vi "MULT_Amostragem_IceMen_FI.vi"(0 "3458A Master":string="22") -> ()   [LabVIEW 2014]
panel:
  out "f":dbl format="%#_8g"
  out "Phase Diff DMM1-DMM2(sec)":dbl[](graph)
  out "FFT":dbl[][](graph)
  out "Phase Diff(sec)":dbl format="%#_10p"
  out "Waveform Graph":dbl[][](graph)
  out "data 2":string
  in  "SLAVE":path=path "C:/Users/diele/Desktop/medição master-slave/SLAVE.txt"
  out "error out 2":errorcluster
  out "OLA EU SOU SLAVE:":string
  in  "3458A Slave":string="3"
  in  "Atraso":i32(ring)=1 items=["", "Inteiro", "Fracionário"]
  in  "Filtro LF":bool
  out "data":string
  out "Abertura (s)":dbl=170.0 min=0.1 max=500.0 step=0.1 format="%#_4g"
  out "V RMS":dbl format="%#_10g"
  out "Delay":dbl=0.10000000149011612 min=0.10000000149011612 max=10000.0 step=0.10000000149011612 format="%.7f"
  out "Harmonicos Medidos":i32
  out "FREQUÊNCIA":dbl format="%#_10g"
  out "Número de Amostras":i32
  out "Intervalo de Amostragem (s)":dbl format="%_10g"
  in  "Número de Harmônicos":i32=50 min=0 max=200 step=1
  out "Iterações":i32
  in  "MASTER":path=path "C:/Users/diele/Desktop/medição master-slave/MASTER.txt"
  in  "NÚMERO DE TRENS DE AMOSTRA":i32=100 min=1 max=1000 step=1
  out "error out":errorcluster
  out "OLA EU SOU MASTER:":string
  # "Aquisição de sinais em baixa frequência através de amostragem digital."
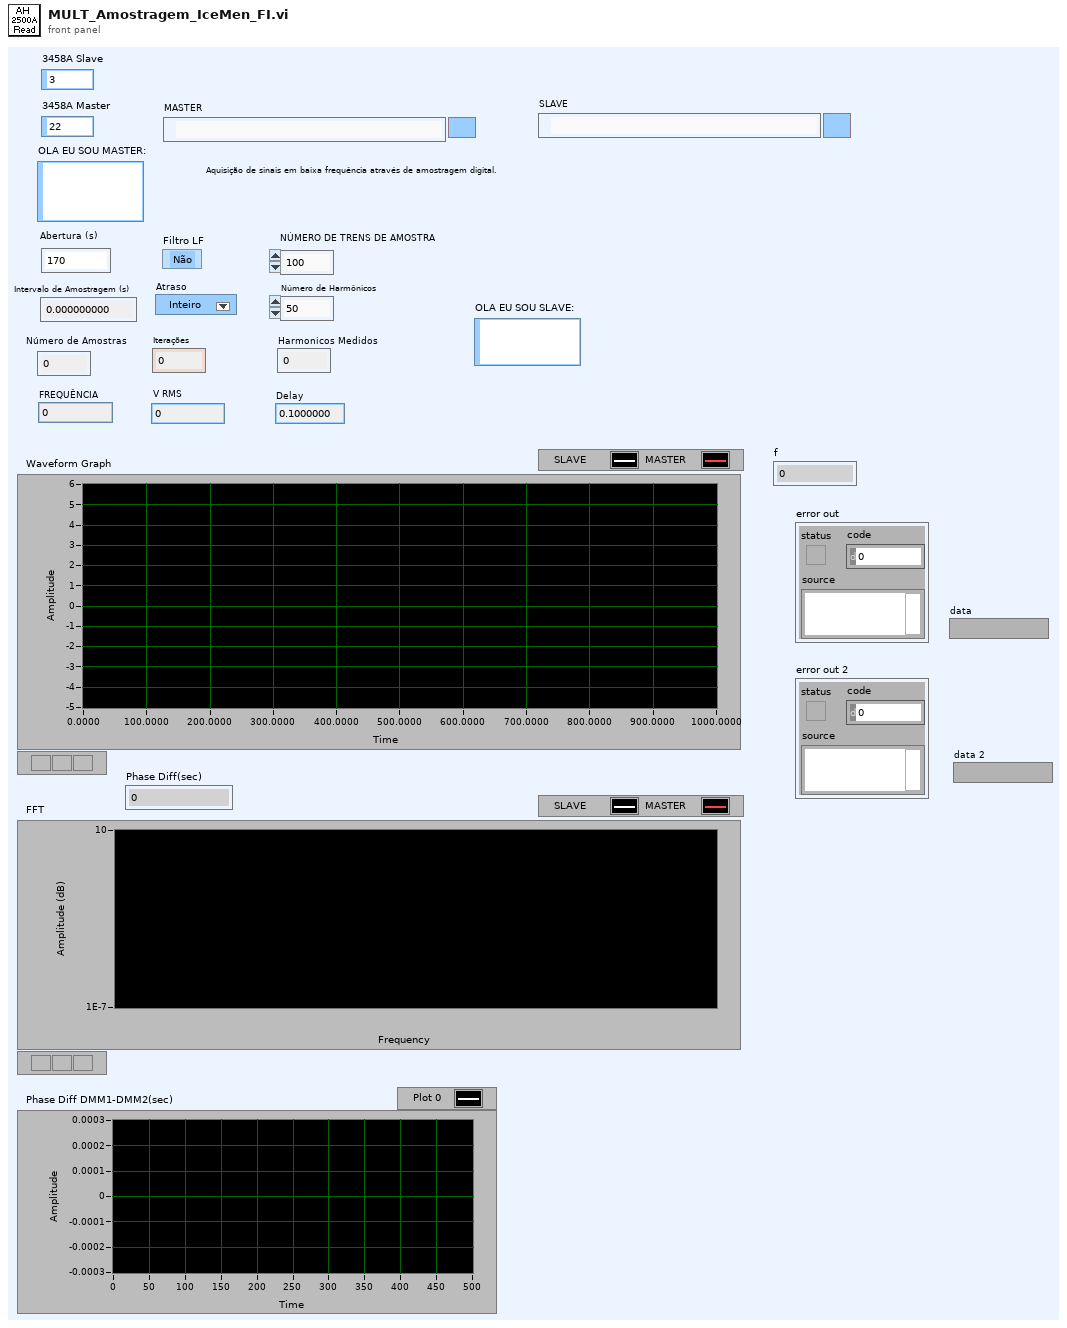
[diagram p1: front panel]
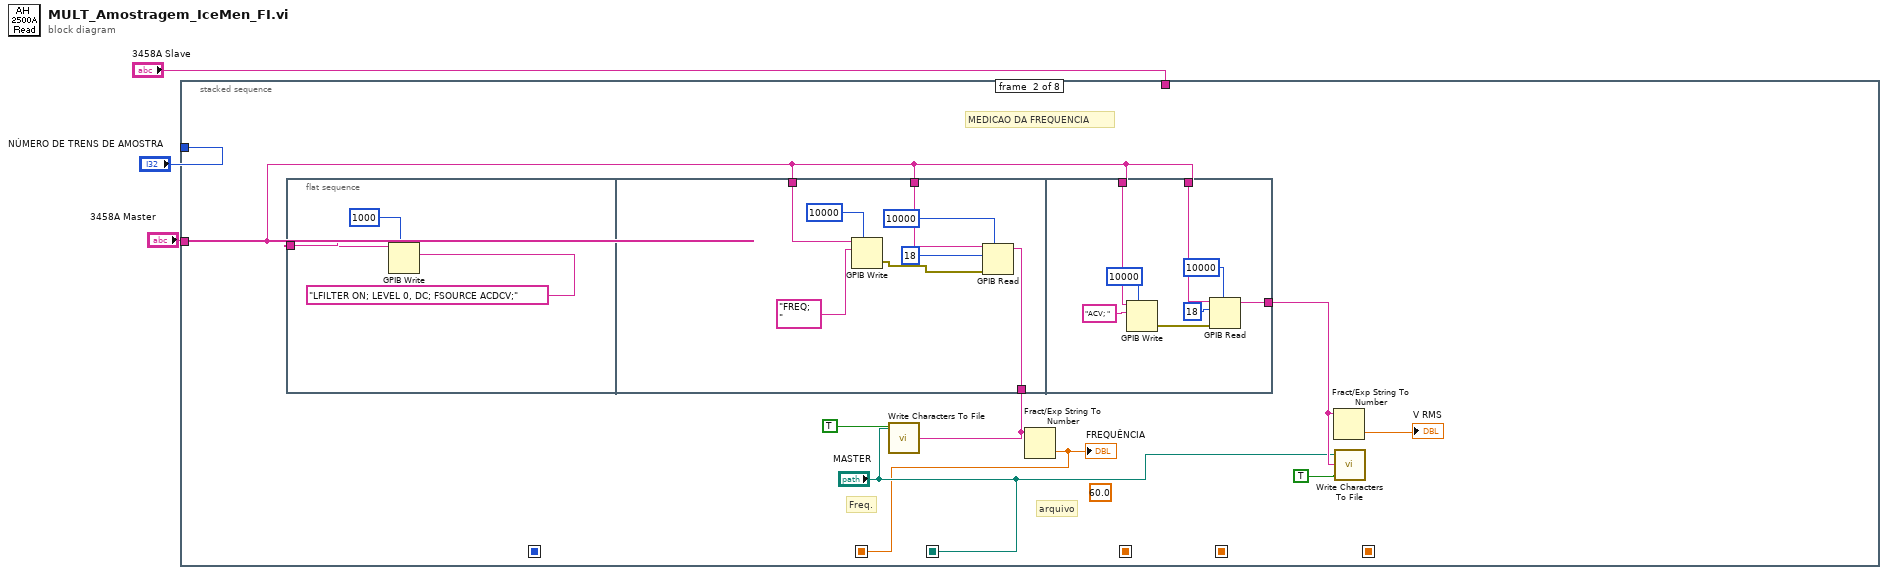
[diagram p0: block diagram]
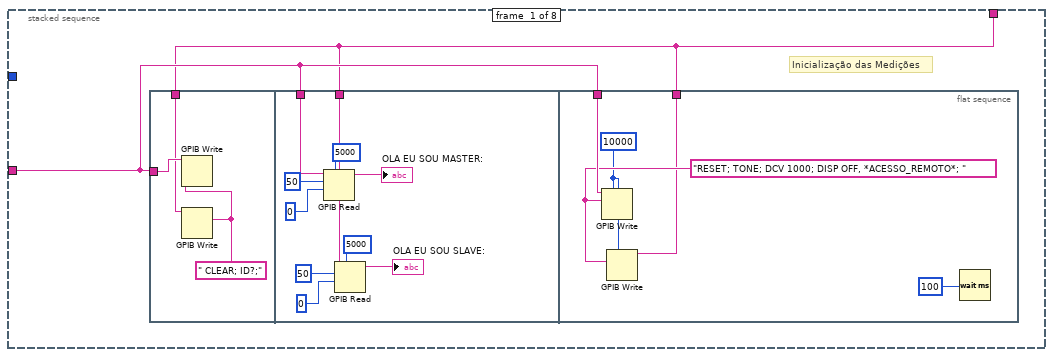
[diagram p2: hidden frame]
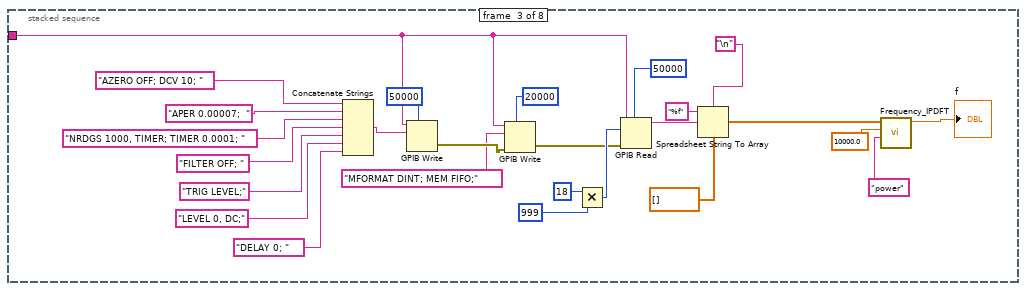
[diagram p3: hidden frame]
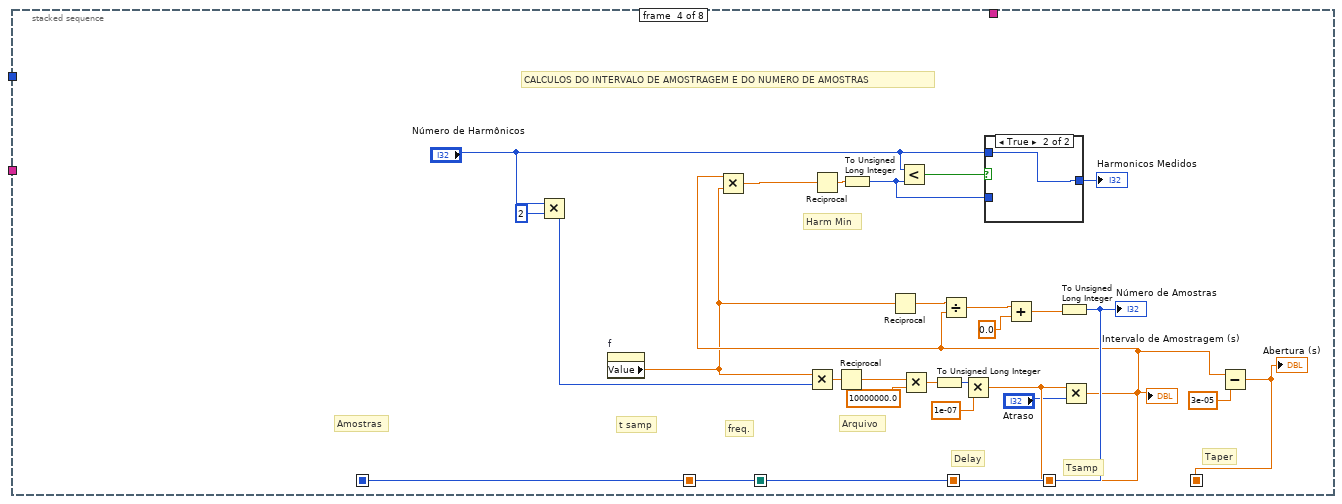
[diagram p4: hidden frame]
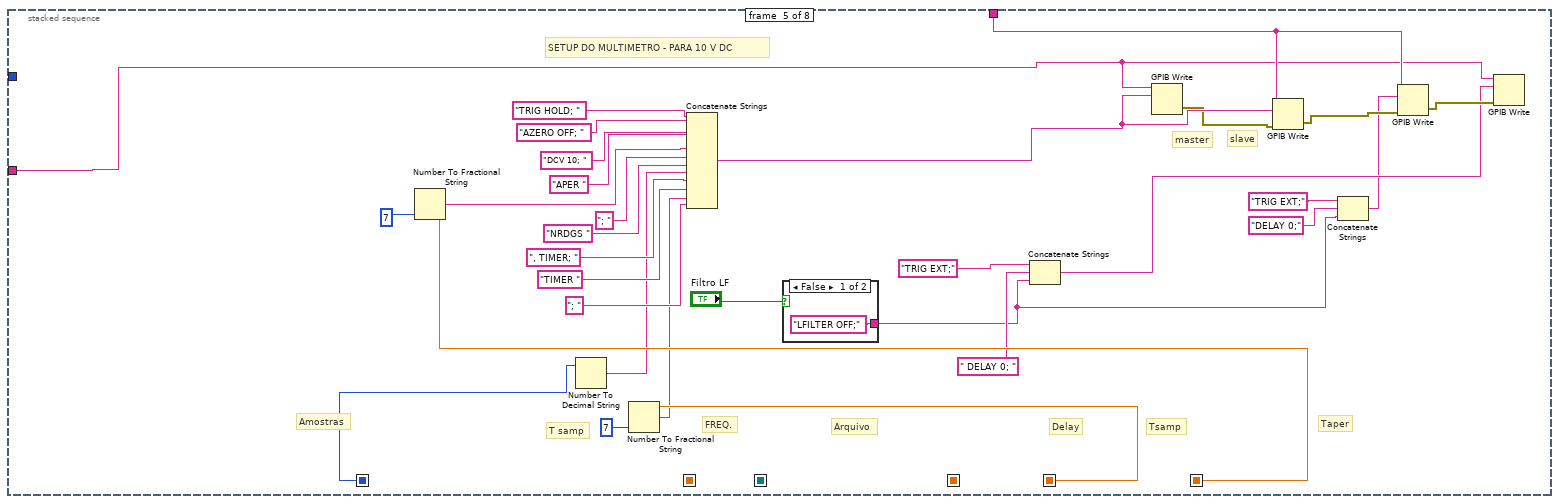
[diagram p6: hidden frame]
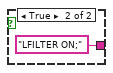
[diagram p7: hidden frame]
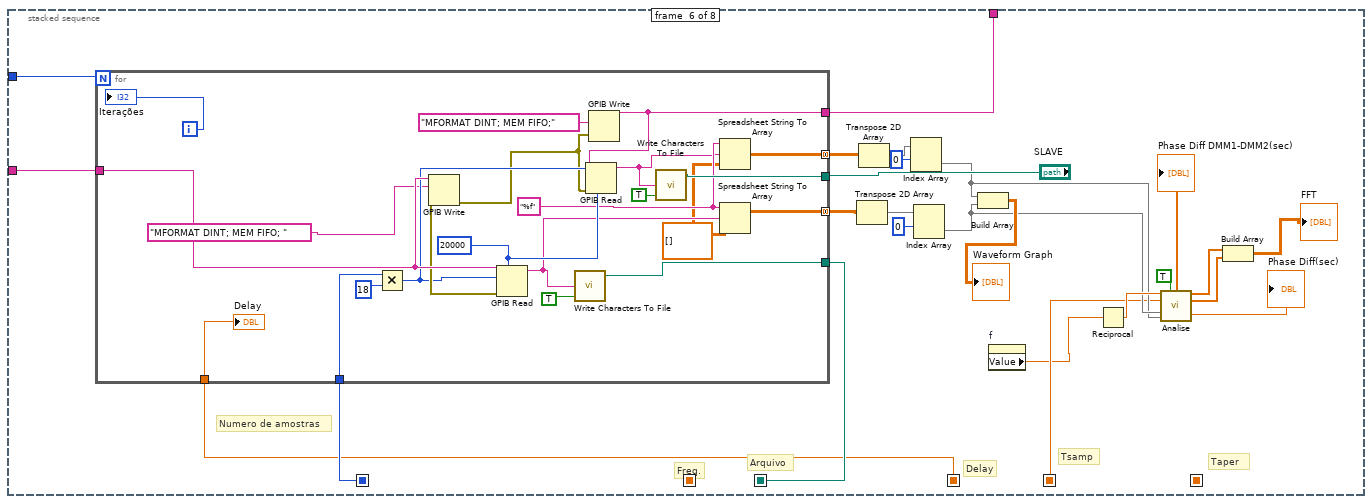
[diagram p8: hidden frame]
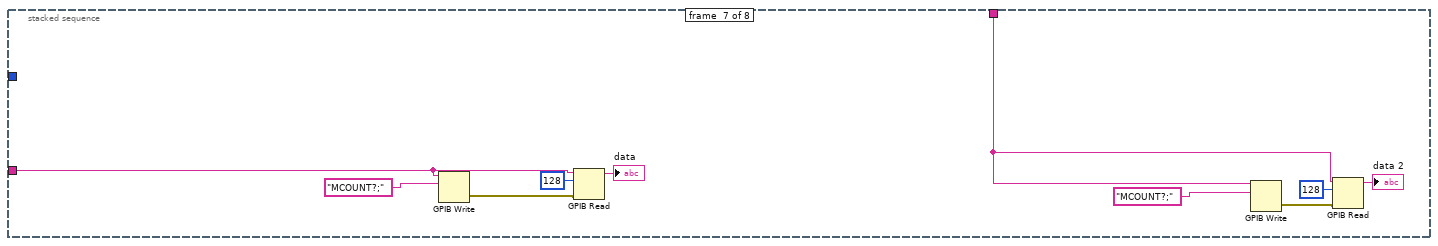
[diagram p9: hidden frame]
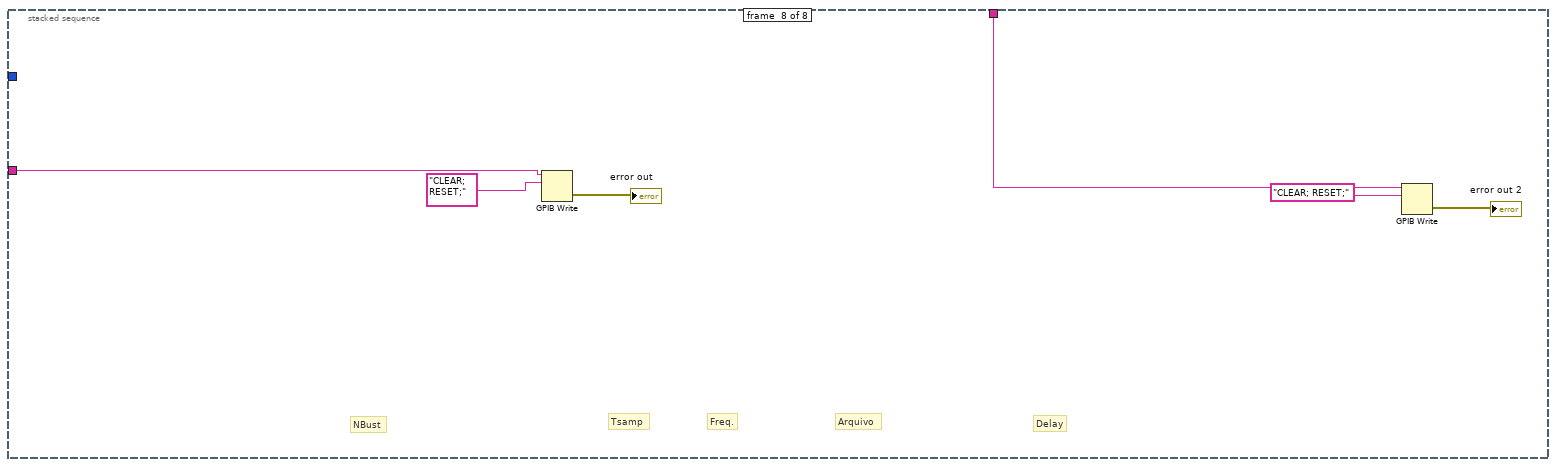
[diagram p10: hidden frame]
diagram:
  n1 = stacked-sequence {
    seq-local: [_ w25 _ _ _ _ _ _] -> [_ _ _ _ _ _ _ _]
    seq-local: [_ _ _ w92 _ _ _ _] -> [_ _ _ _ w123 w161 _ _]
    seq-local: [_ _ _ w80 _ _ _ _] -> [_ _ _ _ w128 w139 _ _]
    seq-local: [_ "MASTER" _ _ _ _ _ _] -> [_ _ _ _ _ w159 _ _]
    seq-local: [_ _ _ w85 _ _ _ _] -> [_ _ _ _ _ w157 _ _]
    seq-local: [_ _ _ w78 _ _ _ _] -> [_ _ _ _ w118 _ _ _]
    tunnel: "3458A Master" -> [w5 w30 w58 _ w111 w160 w191 w198]
    tunnel: "NÚMERO DE TRENS DE AMOSTRA" -> [_ _ _ _ _ w158 _ _]
    tunnel: "3458A Slave" -> [w4 _ _ _ w112 w155 w184 w194]
    frame #0 {
      # "Inicialização das Medições"
      n2 = flat-sequence {
        tunnel: w5 -> [w8]
        tunnel: w4 -> [w7]
        tunnel: w5 -> [w14]
        tunnel: w4 -> [w9]
        tunnel: w5 -> [w23]
        tunnel: w4 -> [w20]
        frame #0 {
          w6 = " CLEAR; ID?;" ("data")
          n3 = GPIB Write(0:w8, 1:w6) -> ()  [unwired: 3 in, 2 out]
          n4 = GPIB Write(0:w7, 1:w6) -> ()  [unwired: 3 in, 2 out]
        }
        frame #1 {
          n5 = GPIB Read(0:w14, 1:50, 2:i16 0, 4:5000 ("timeout ms (488.2 global)")) -> (5:→"OLA EU SOU MASTER:":string)  [unwired: 1 in, 2 out]
          n6 = GPIB Read(0:w9, 1:50, 2:i16 0, 4:5000 ("timeout ms (488.2 global)")) -> (5:→"OLA EU SOU SLAVE:":string)  [unwired: 1 in, 2 out]
        }
        frame #2 {
          w19 = 10000 ("timeout ms (488.2 global)")
          w21 = "RESET; TONE; DCV 1000; DISP OFF, *ACESSO_REMOTO*; " ("data")
          n7 = GPIB Write(0:w23, 1:w21, 4:w19) -> ()  [unwired: 2 in, 2 out]
          n8 = GPIB Write(0:w20, 1:w21, 4:w19) -> ()  [unwired: 2 in, 2 out]
          n9 = Wait (ms)(milliseconds to wait=u32 100) -> ()  [unwired: 1 out]
        }
      }
    }
    frame #1 {
      (unwired) 60.0
      # "Freq."
      # "arquivo"
      # "MEDICAO DA FREQUENCIA"
      n10 = flat-sequence {
        tunnel: w30 -> [w34]
        tunnel: w30 -> [w42]
        tunnel: w30 -> [w39]
        tunnel: [w35] -> w31
        tunnel: w30 -> [w45]
        tunnel: w30 -> [w44]
        tunnel: [w43] -> w28
        frame #0 {
          n11 = GPIB Write(0:w34, 1:"LFILTER ON; LEVEL 0, DC; FSOURCE ACDCV;", 4:1000 ("timeout ms (488.2 global)")) -> ()  [unwired: 2 in, 2 out]
        }
        frame #1 {
          n12 = GPIB Write(0:w42, 1:"FREQ;  ", 4:10000 ("timeout ms (488.2 global)")) -> (6:w36:errorcluster)  [unwired: 2 in, 1 out]
          n13 = GPIB Read(0:w39, 1:18 ("byte count"), 3:w36, 4:10000 ("timeout ms (488.2 global)")) -> (5:w35:string)  [unwired: 1 in, 2 out]
        }
        frame #2 {
          n14 = GPIB Write(0:w45, 1:"ACV; ", 4:10000 ("timeout ms (488.2 global)")) -> (6:w46:errorcluster)  [unwired: 2 in, 1 out]
          n15 = GPIB Read(0:w44, 1:18 ("byte count"), 3:w46, 4:10000 ("timeout ms (488.2 global)")) -> (5:w43:string)  [unwired: 1 in, 2 out]
        }
      }
      n16 = call <vilib>:"Write Characters To File.vi"("append to file? (new file:F)"=TRUE, "character string"=w31, "file path (dialog if empty)"="MASTER") -> ()  [unwired: 2 in, 1 out]
      n17 = Fract/Exp String To Number(string=w31) -> (number=w25:dbl)  [unwired: 3 in, 1 out]
      "FREQUÊNCIA" <- w25
      n18 = Fract/Exp String To Number(string=w28) -> (number=→"V RMS":dbl)  [unwired: 3 in, 1 out]
      n19 = call <vilib>:"Write Characters To File.vi"("append to file? (new file:F)"=TRUE ("transpose? (no:F)"), "character string"=w28, "file path (dialog if empty)"="MASTER") -> ()  [unwired: 2 in, 1 out]
    }
    frame #2 {
      n20 = Concatenate Strings("AZERO OFF; DCV 10; ", "APER 0.00007;  " ("string"), "NRDGS 1000, TIMER; TIMER 0.0001; ", "FILTER OFF; " ("string"), "TRIG LEVEL;" ("string"), "LEVEL 0, DC;" ("string"), "DELAY 0; " ("string")) -> (w70:string)
      n21 = GPIB Write(0:w58, 1:w70, 4:50000 ("timeout ms (488.2 global)")) -> (6:w59:errorcluster)  [unwired: 2 in, 1 out]
      n22 = GPIB Write(0:w58, 1:"MFORMAT DINT; MEM FIFO;" ("data"), 3:w59, 4:20000 ("timeout ms (488.2 global)")) -> (6:w57:errorcluster)  [unwired: 1 in, 1 out]
      n23 = Multiply(x=18 ("byte count"), y=999) -> (x*y=w61:i32)
      n24 = GPIB Read(0:w58, 1:w61, 3:w57, 4:50000 ("timeout ms (488.2 global)")) -> (5:w74:string)  [unwired: 1 in, 2 out]
      n25 = Spreadsheet String To Array(delimiter (Tab)="\n", format string="%f", spreadsheet string=w74, array type (2D Dbl)=dbl[] []) -> (array=w73:dbl[])
      n26 = call "Frequency_IPDFT.vi"("Estimation Model"="power", "Fs"=10000.0, "Signal"=w73) -> ("f"=→"f":dbl)  [unwired: 8 in]
    }
    frame #3 {
      # "Taper"
      # "Amostras"
      # "Arquivo"
      # "t samp"
      # "Delay"
      # "Harm Min"
      # "freq."
      # "Tsamp"
      # "CALCULOS DO INTERVALO DE AMOSTRAGEM E DO NUMERO DE AMOSTRAS"
      n27 = Multiply(x="Número de Harmônicos", y=2) -> (x*y=w81:i32)
      n28 = property on="f" class="DigNum (strict)"() -> ("Value"=w77:dbl)  [unwired: 2 in, 2 out]
      n29 = Multiply(x=w77, y=w81) -> (x*y=w91:dbl)
      n30 = Reciprocal(x=w91) -> (1/x=w86:dbl)
      n31 = Reciprocal(x=w77) -> (1/x=w96:dbl)
      n32 = Multiply(x=w86, y=10000000.0) -> (x*y=w89:dbl)
      n33 = To Unsigned Long Integer(number=w89) -> (unsigned 32bit integer=w88:u32)
      n34 = Multiply(x=w88, y=1e-07) -> (x*y=w85:dbl)
      n35 = Multiply(x=w85, y="Atraso") -> (x*y=w80:dbl)
      "Intervalo de Amostragem (s)" <- w80
      n36 = Multiply(x=w80, y=w77) -> (x*y=w101:dbl)
      n37 = Reciprocal(x=w101) -> (1/x=w100:dbl)
      n38 = To Unsigned Long Integer(number=w100) -> (unsigned 32bit integer=w97:u32)
      n39 = Less?(x="Número de Harmônicos", y=w97) -> (x < y?=w99:bool)
      n40 = Divide(x=w96, y=w80) -> (x/y=w95:dbl)
      n41 = case shown="True" w99 {
        tunnel: [w102 w103] -> w98
        tunnel: "Número de Harmônicos" -> [_ w103]
        tunnel: w97 -> [w102 _]
        frame False {
        }
        frame True {
        }
      }
      "Harmonicos Medidos" <- w98
      n42 = Add(x=w95, y=0.0) -> (x+y=w93:dbl)
      n43 = To Unsigned Long Integer(number=w93) -> (unsigned 32bit integer=w92:u32)
      "Número de Amostras" <- w92
      n44 = Subtract(x=w80, y=3e-05) -> (x-y=w78:dbl)
      "Abertura (s)" <- w78
    }
    frame #4 {
      # "master"
      # "slave"
      # "Taper"
      # "Tsamp"
      # "Delay"
      # "Arquivo"
      # "Amostras"
      # "T samp"
      # "FREQ."
      # "SETUP DO MULTIMETRO - PARA 10 V DC"
      n45 = Number To Fractional String(number=w118, precision (6)=i16 7) -> (F-format string=w130:string)  [unwired: 2 in]
      n46 = Number To Decimal String(number=w123) -> (decimal integer string=w117:string)  [unwired: 1 in]
      n47 = Number To Fractional String(number=w128, precision (6)=i16 7) -> (F-format string=w116:string)  [unwired: 2 in]
      n48 = Concatenate Strings("TRIG HOLD; ", "AZERO OFF; ", "DCV 10; ", "APER " ("string"), w130, "; " ("string"), "NRDGS ", w117, ", TIMER; " ("string"), "TIMER " ("string"), w116, "; " ("string")) -> (w115:string)
      n49 = case shown="False" "Filtro LF" {
        tunnel: ["LFILTER OFF;" ("string") "LFILTER ON;" ("string")] -> w104
        frame False {
        }
        frame True {
        }
      }
      n50 = Concatenate Strings("TRIG EXT;" ("string"), " DELAY 0; " ("string"), w104) -> (w107:string)
      n51 = GPIB Write(0:w111, 1:w115) -> (6:w108:errorcluster)  [unwired: 3 in, 1 out]
      n52 = GPIB Write(0:w112, 1:w115, 3:w108) -> (6:w110:errorcluster)  [unwired: 2 in, 1 out]
      n53 = Concatenate Strings("TRIG EXT;" ("string"), "DELAY 0;" ("string"), w104) -> (w106:string)
      n54 = GPIB Write(0:w112, 1:w106, 3:w110) -> (6:w109:errorcluster)  [unwired: 2 in, 1 out]
      n55 = GPIB Write(0:w111, 1:w107, 3:w109) -> ()  [unwired: 2 in, 2 out]
    }
    frame #5 {
      # "Taper"
      # "Delay"
      # "Freq."
      # "Arquivo"
      # "Numero de amostras"
      # "Tsamp"
      n56 = for {
        N: w158 -> [_]
        tunnel: w161 -> [w176]
        tunnel: w160 -> [w181]
        tunnel: w159 -> [w179]
        tunnel: w157 -> [w178]
        tunnel: "SLAVE" -> [w174]
        tunnel: w155 -> [w175]
        tunnel: [w170] -> w154 mode=concatenating
        tunnel: [w165] -> w153 mode=concatenating
        i -> [w177]
        w167 = dbl[][] [] ("array type (2D Dbl)")
        w168 = "%f" ("format string")
        w171 = 20000 ("timeout ms (488.2 global)")
        n57 = Multiply(x=w176, y=18) -> (x*y=w172:u32)
        n58 = GPIB Write(0:w175, 1:"MFORMAT DINT; MEM FIFO;" ("data")) -> (6:w163:errorcluster)  [unwired: 3 in, 1 out]
        n59 = GPIB Write(0:w181, 1:"MFORMAT DINT; MEM FIFO; " ("string"), 3:w163) -> (6:w180:errorcluster)  [unwired: 2 in, 1 out]
        n60 = GPIB Read(0:w181, 1:w172, 3:w180, 4:w171) -> (5:w169:string)  [unwired: 1 in, 2 out]
        n61 = call <vilib>:"Write Characters To File.vi"("append to file? (new file:F)"=TRUE ("transpose? (no:F)"), "character string"=w169, "file path (dialog if empty)"=w179) -> ()  [unwired: 2 in, 1 out]
        n62 = GPIB Read(0:w175, 1:w172, 3:w163, 4:w171) -> (5:w166:string)  [unwired: 1 in, 2 out]
        n63 = call <vilib>:"Write Characters To File.vi"("append to file? (new file:F)"=TRUE, "character string"=w166, "file path (dialog if empty)"=w174) -> ()  [unwired: 2 in, 1 out]
        n64 = Spreadsheet String To Array(format string=w168, spreadsheet string=w166, array type (2D Dbl)=w167) -> (array=w165:dbl[][])  [unwired: 1 in]
        n65 = Spreadsheet String To Array(format string=w168, spreadsheet string=w169, array type (2D Dbl)=w167) -> (array=w170:dbl[][])  [unwired: 1 in]
        "Delay" <- w178
        "Iterações" <- w177
      }
      n66 = Transpose 2D Array(2D array=w154) -> (transposed array=w150:dbl[][])
      n67 = Transpose 2D Array(2D array=w153) -> (transposed array=w152:dbl[][])
      n68 = Index Array(array=w152, index (row)=0) -> (element=w140:dbl[])  [unwired: 1 in]
      n69 = Index Array(array=w150, index (row)=0) -> (element=w141:dbl[])  [unwired: 1 in]
      n70 = Build Array(w140, w141) -> (→"Waveform Graph":dbl[][])
      n71 = property on="f" class="DigNum (strict)"() -> ("Value"=w137:dbl)  [unwired: 2 in, 2 out]
      n72 = Reciprocal(x=w137) -> (1/x=w142:dbl)
      n73 = call "Analise.vi"("Período"=w142, "Análise"=TRUE, "Tempo entre amostras"=w139, "DMM1"=w141, "DMM2"=w140) -> ("Phase Diff DMM1-DMM2(sec)"=→"Phase Diff DMM1-DMM2(sec)":dbl[], "Amplitude DMM 1"=w145:dbl[], "Amplitude DMM 2"=w146:dbl[], "Phase Diff(sec)"=→"Phase Diff(sec)":dbl)  [unwired: 1 in, 6 out]
      n74 = Build Array(w145, w146) -> (→"FFT":dbl[][])
    }
    frame #6 {
      n75 = GPIB Write(0:w191, 1:"MCOUNT?;" ("data")) -> (6:w192:errorcluster)  [unwired: 3 in, 1 out]
      n76 = GPIB Read(0:w191, 1:128 ("byte count"), 3:w192) -> (5:→"data":string)  [unwired: 2 in, 2 out]
      n77 = GPIB Write(0:w184, 1:"MCOUNT?;" ("data")) -> (6:w187:errorcluster)  [unwired: 3 in, 1 out]
      n78 = GPIB Read(0:w184, 1:128 ("byte count"), 3:w187) -> (5:→"data 2":string)  [unwired: 2 in, 2 out]
    }
    frame #7 {
      # "Delay"
      # "Freq."
      # "Tsamp"
      # "Arquivo"
      # "NBust"
      n79 = GPIB Write(0:w198, 1:"CLEAR; RESET;" ("data")) -> (6:→"error out":errorcluster)  [unwired: 3 in, 1 out]
      n80 = GPIB Write(0:w194, 1:"CLEAR; RESET;" ("data")) -> (6:→"error out 2":errorcluster)  [unwired: 3 in, 1 out]
    }
  }
